vi "IdleState.vi"(8 "error in (no error)":errorcluster, 9 "Cluster in":T2, 10 "Enum in":T1, 11 "Actual Start [i]":i64) -> (0 "error out":errorcluster, 2 "Cluster out":T2, 3 "Enum":T1)   [LabVIEW 2018]
uses:
  Type_Def/Type_Def Actuator Controls.ctl
  Type_Def/Type_Def ControlState.ctl
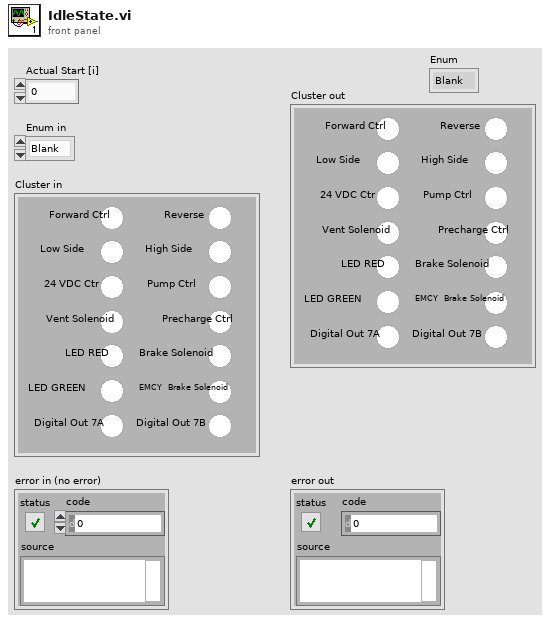
[diagram p1: front panel]
types:
  T1 = typedef "Type_Def ControlState.ctl" = enum16{"Blank", "Systems Check", "Idle", "Ready", "Pushing", "CrawlingPrecharge", "Braking", "Fault", "Boot Up", "Crawling", "Shutdown", "Service Push", "Service Wait", "Vent", "Precharge"}
  T2 = typedef "Type_Def Actuator Controls.ctl" = cluster{"Reverse ":bool, "Precharge Ctrl":bool, "Pump Ctrl":bool, "24 VDC Ctr":bool, "Vent Solenoid":bool, "Brake Solenoid":bool, "EMCY  Brake Solenoid":bool, "Digital Out 7B ":bool, "Forward Ctrl":bool, " Low Side":bool, "High Side":bool, "LED RED":bool, "LED GREEN":bool, " Digital Out 7A":bool}
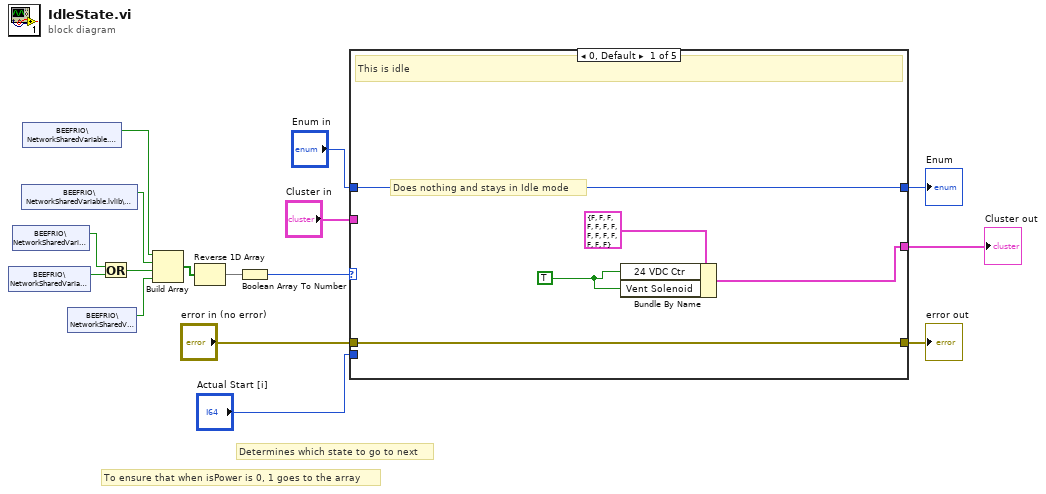
[diagram p0: block diagram]
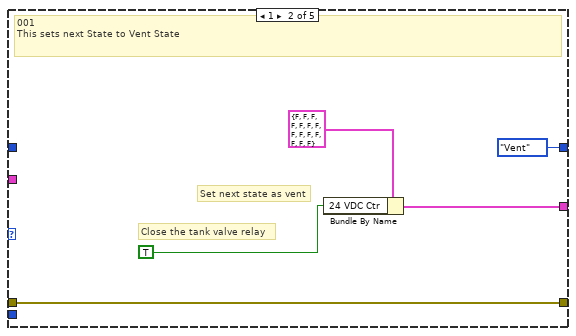
[diagram p2: hidden frame]
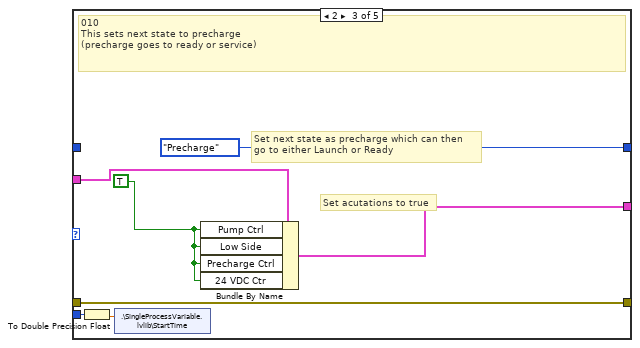
[diagram p3: hidden frame]
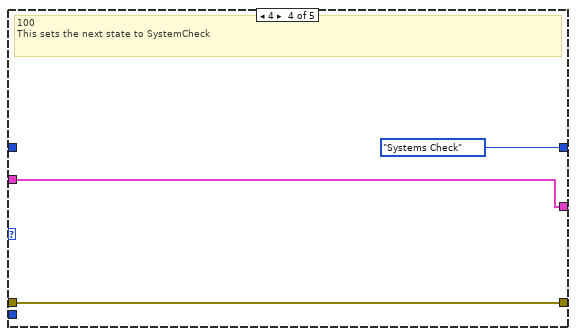
[diagram p4: hidden frame]
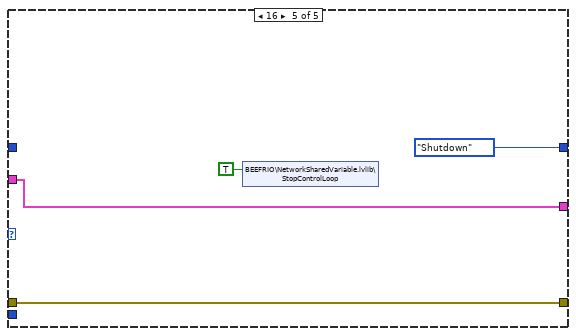
[diagram p5: hidden frame]
diagram:
  # "To ensure that when isPower is 0, 1 goes to the array"
  # "Determines which state to go to next"
  n1 = shared-variable "BEEFRIO\\NetworkSharedVariable.lvlib\\Service"() -> (w11:bool)  [unwired: 1 in, 1 out]
  n2 = shared-variable "BEEFRIO\\NetworkSharedVariable.lvlib\\Ready"() -> (w12:bool)  [unwired: 1 in, 1 out]
  n3 = shared-variable "BEEFRIO\\NetworkSharedVariable.lvlib\\SystemCheck"() -> (w2:bool)  [unwired: 1 in, 1 out]
  n4 = shared-variable "BEEFRIO\\NetworkSharedVariable.lvlib\\Shutdown"() -> (w1:bool)  [unwired: 1 in, 1 out]
  n5 = shared-variable "BEEFRIO\\NetworkSharedVariable.lvlib\\Vent"() -> (w7:bool)  [unwired: 1 in, 1 out]
  n6 = Or(x=w12, y=w11) -> (x .or. y?=w13:bool)
  n7 = Build Array(w1, w2, w13, w7) -> (w8:bool[])
  n8 = Reverse 1D Array(array=w8) -> (reversed array=w9:bool[])
  n9 = Boolean Array To Number(Boolean array=w9) -> (number=w10:u32)
  n10 = case shown="0, Default" w10 {
    tunnel: "Enum in" -> [w21 _ _ _ _]
    tunnel: [w21 Type_Def_ControlState."Vent" Type_Def_ControlState."Precharge" Type_Def_ControlState."Systems Check" Type_Def_ControlState."Shutdown" ("Enum in")] -> w4
    tunnel: "Cluster in" -> [_ _ w32 w35 w40]
    tunnel: [w18 w24 w31 w35 w40] -> w6
    tunnel: [w20 w23 w30 w34 w38] -> w14
    tunnel: "error in (no error)" -> [w20 w23 w30 w34 w38]
    tunnel: "Actual Start [i]" -> [_ _ w29 _ _]
    frame 0, Default {
      w17 = TRUE ("24 VDC Ctr")
      # "Does nothing and stays in Idle mode"
      # "This is idle"
      n11 = Bundle By Name(cluster=T2 {"Reverse "=FALSE, "Precharge Ctrl"=FALSE, "Pump Ctrl"=FALSE, "24 VDC Ctr"=FALSE, "Vent Solenoid"=FALSE, "Brake Solenoid"=FALSE, "EMCY  Brake Solenoid"=FALSE, "Digital Out 7B "=FALSE, "Forward Ctrl"=FALSE, " Low Side"=FALSE, "High Side"=FALSE, "LED RED"=FALSE, "LED GREEN"=FALSE, " Digital Out 7A"=FALSE} ("Cluster in 2"), "24 VDC Ctr"=w17, "Vent Solenoid"=w17) -> (w18:T2)
    }
    frame 1 {
      # "Set next state as vent"
      # "Close the tank valve relay"
      # "001\nThis sets next State to Vent State"
      n12 = Bundle By Name(cluster=T2 {"Reverse "=FALSE, "Precharge Ctrl"=FALSE, "Pump Ctrl"=FALSE, "24 VDC Ctr"=FALSE, "Vent Solenoid"=FALSE, "Brake Solenoid"=FALSE, "EMCY  Brake Solenoid"=FALSE, "Digital Out 7B "=FALSE, "Forward Ctrl"=FALSE, " Low Side"=FALSE, "High Side"=FALSE, "LED RED"=FALSE, "LED GREEN"=FALSE, " Digital Out 7A"=FALSE} ("Cluster in 2"), "24 VDC Ctr"=TRUE) -> (w24:T2)
    }
    frame 2 {
      w27 = TRUE
      # "Set next state as precharge which can then \ngo to either Launch or Ready"
      # "Set acutations to true"
      # "010\nThis sets next state to precharge \n(precharge goes to ready or service)"
      n13 = To Double Precision Float(number=w29) -> (double precision float=w28:dbl)
      n14 = shared-variable ".\\SingleProcessVariable.lvlib\\StartTime"(w28) -> ()  [unwired: 1 in, 1 out]
      n15 = Bundle By Name(cluster=w32, "Pump Ctrl"=w27, "Low Side"=w27, "Precharge Ctrl"=w27, "24 VDC Ctr"=w27) -> (w31:T2)
    }
    frame 4 {
      # "100\nThis sets the next state to SystemCheck"
    }
    frame 16 {
      n16 = shared-variable "BEEFRIO\\NetworkSharedVariable.lvlib\\StopControlLoop"(TRUE ("StopControlLoop")) -> ()  [unwired: 1 in, 1 out]
    }
  }
  "error out" <- w14
  "Cluster out" <- w6
  "Enum" <- w4
